vi "I2C start.vi"   [LabVIEW 2019]
uses:
  <vilib>/rvi/eio/common/nirviEmuTemplateMethod_errors.vi
  <vilib>/eio/EIONode/EIONode.xnode
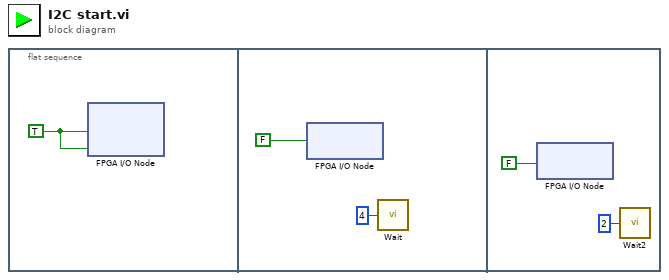
[diagram p0: block diagram]
diagram:
  n1 = flat-sequence {
    frame #0 {
      w1 = TRUE
      n2 = xnode "FPGA I/O Node"("SDA"=w1, "SCL"=w1) -> ()  [unwired: 2 in, 2 out]
    }
    frame #1 {
      n3 = xnode "FPGA I/O Node"("SDA"=FALSE ("ConnectorA/DIO15")) -> ()  [unwired: 1 in, 1 out]
      n4 = call "Wait"("Count(uSec)"=u32 4) -> ()  [unwired: 1 out]
    }
    frame #2 {
      n5 = xnode "FPGA I/O Node"("SCL"=FALSE ("ConnectorA/DIO14")) -> ()  [unwired: 1 in, 1 out]
      n6 = call "Wait2"("Count(uSec)"=u32 2) -> ()  [unwired: 1 out]
    }
  }
